vi "Launch Actor.vi"   [LabVIEW 2023]
uses:
  Host MSS Test Actor/Host MSS Test Actor.lvclass
  C:/Program Files/National Instruments/LabVIEW 2023/vi.lib/ActorFramework/Actor/Actor.lvclass
  <vilib>/ni/Actors/Network Endpoint Actors/Protocols/Network Stream Strategy/Network Stream/Network Stream.lvclass/Network Stream.ctl
  <vilib>/ni/Actors/Network Endpoint Actors/Protocols/Network Stream Strategy/Network Stream Initiator/Network Stream Initiator.lvclass/Network Stream Initiator.ctl
  Host MSS Test Actor/Host MSS Test Actor.lvclass/Host MSS Test Actor.ctl
  <vilib>/ni/Actors/Network Endpoint Actors/Protocols/Network Stream Strategy/Network Stream/Write Buffer Size.vi
  <vilib>/ni/Actors/Network Endpoint Actors/Protocols/Network Stream Strategy/Network Stream/Write Name.vi
  <vilib>/ni/Actors/Network Endpoint Actors/Protocols/Network Stream Strategy/Network Stream Initiator/Network Stream Initiator.lvclass
  C:/Program Files/National Instruments/LabVIEW 2023/vi.lib/ni/Actors/Network Endpoint Actors/Protocols/Network Stream Strategy/Network Stream/Network Stream.lvclass
  C:/Program Files/National Instruments/LabVIEW 2023/vi.lib/ni/Actors/Network Endpoint Actors/Abstract Classes/Message Stream/Message Stream.lvclass
  <vilib>/ni/Actors/Network Endpoint Actors/Protocols/Network Stream Strategy/Network Stream/Write Address.vi
  <vilib>/ActorFramework/Actor/Actor.lvclass
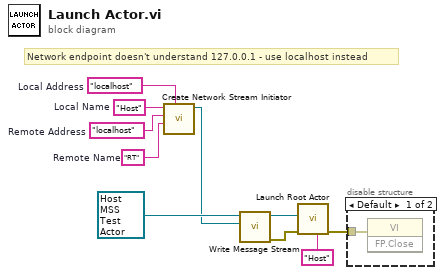
[diagram p0: block diagram]
diagram:
  w9 = "RT"  # Remote Name
  w8 = "localhost"  # Local Address
  w10 = "localhost"  # Remote Address
  w1 = "Host"  # Local Name
  # "Network endpoint doesn't understand 127.0.0.1 - use localhost instead"
  n1 = call <vilib>:"Create Network Stream Initiator.vi"("Local Address"=w8, "Remote Name"=w9, "Remote Address"=w10, "Name"=w1) -> ("Network Stream Initiator out"=w4:refnum<class "Network Stream Initiator.lvclass">)  [unwired: 7 in]
  n2 = call "Write Message Stream.vi"("Message Stream.lvclass"=w4, "Host MSS Test Actor in"=refnum<class "Host MSS Test Actor.lvclass"> refnum ("Host MSS Test Actor.lvlib:Host MSS Test Actor.lvclass")) -> ("error out"=w7:errorcluster, "Host MSS Test Actor out"=w5:refnum<class "Host MSS Test Actor.lvclass">)  [unwired: 8 in]
  n3 = call <vilib>:"Launch Root Actor.vi"("Debug Alias"="Host", "error in (no error)"=w7, "Actor"=w5) -> ("error out"=w3:errorcluster)  [unwired: 7 in, 1 out]
  n4 = disable-structure shown="Default" {
    disable-tunnel: w3 -> [w11 _]
    frame condition #0 {
      n5 = invoke class="VI" method="FP.Close"(error in=w11) -> ()  [unwired: 2 in, 3 out]
    }
    frame condition #1 (active) {
    }
  }
